vi "Interpolation Test.vi"() -> ()   [LabVIEW 2014]
uses:
  <vilib>/rvi/interface/nirviMethod/nirviMethod.xnode
  <vilib>/FPGAPlugInAG/Dynamic/niLvFpga_Abort_Dynamic.vi
  <vilib>/rvi/interface/nirviCloseFPGA/nirviCloseFPGA.xnode
  <vilib>/FPGAPlugInAG/Dynamic/niLvFpga_Close_Dynamic.vi
panel:
  in  "stop":bool
  out "Detected Frequency (Hz)":dbl
  in  "Sample Rate (S/s)":dbl=50000000.0 format="%#_13g"
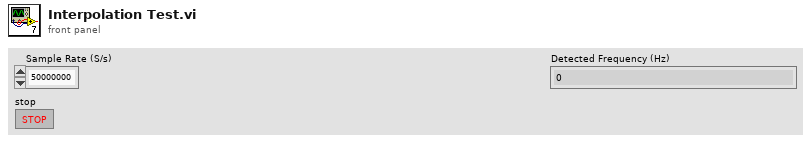
[diagram p1: front panel]
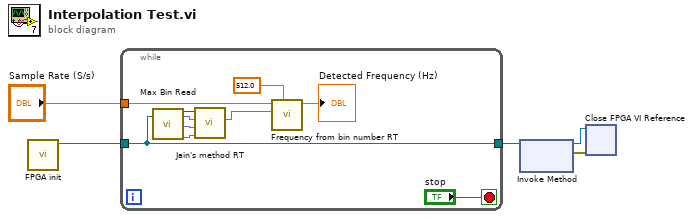
[diagram p0: block diagram]
diagram:
  n1 = call "FPGA init.vi"() -> ("FPGA VI Reference Out"=w5:refnum<k20>)  [unwired: 10 in, 1 out]
  n2 = while {
    tunnel: w5 -> [w10]
    tunnel: "Sample Rate (S/s)" -> [w7]
    tunnel: [w10] -> w3
    stop <- "stop" stop-if-true
    n3 = call "Max Bin Read.vi"("FPGA VI Reference In"=w10) -> ("Max Bin"=w15:i32, "Max Amp"=w14:fxp<+,46,22>, "Next Amp"=w13:fxp<+,46,22>, "Prev Amp"=w12:fxp<+,46,22>)  [unwired: 13 in, 2 out]
    n4 = call "Jain's method RT.vi"("Prev Amp"=w12, "Next Amp"=w13, "Max Amp"=w14, "Max Bin"=w15) -> ("Bin"=w6:fxp<+/-,64,66>)  [unwired: 7 in]
    n5 = call "Frequency from bin number RT.vi"("FFT size"=512.0, "Bin number"=w6, "Sample Rate (S/s)"=w7) -> ("Detected Frequency (Hz)"=→"Detected Frequency (Hz)":dbl)  [unwired: 8 in]
  }
  n6 = xnode "Invoke Method"("FPGA VI Reference In"=w3) -> ("FPGA VI Reference Out"=w2:refnum<k20>, "error out"=w1:errorcluster)  [unwired: 1 in]
  n7 = xnode "Close FPGA VI Reference"("FPGA VI Reference In"=w2, "error in"=w1) -> ()  [unwired: 1 out]
